vi "STS.vi"() -> ()   [LabVIEW 2014]
panel:
  out "Efficiency":dbl
  out "Mechanical Output Power":dbl
  out "Supply power":dbl
  out "Speed":dbl
  out "i":dbl
  in  "Supply Voltage":dbl
  in  "Load Torque":dbl
  # "Ahmed Adel Hassan Elmashhor"
  # "Sec 1"
  # "Steady State Analysis of DC Motor"
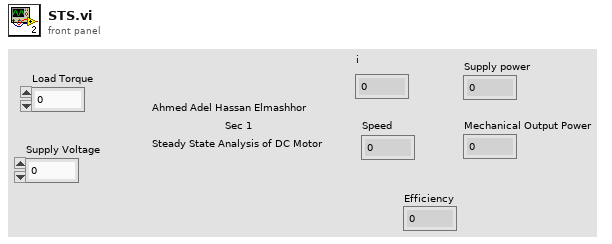
[diagram p1: front panel]
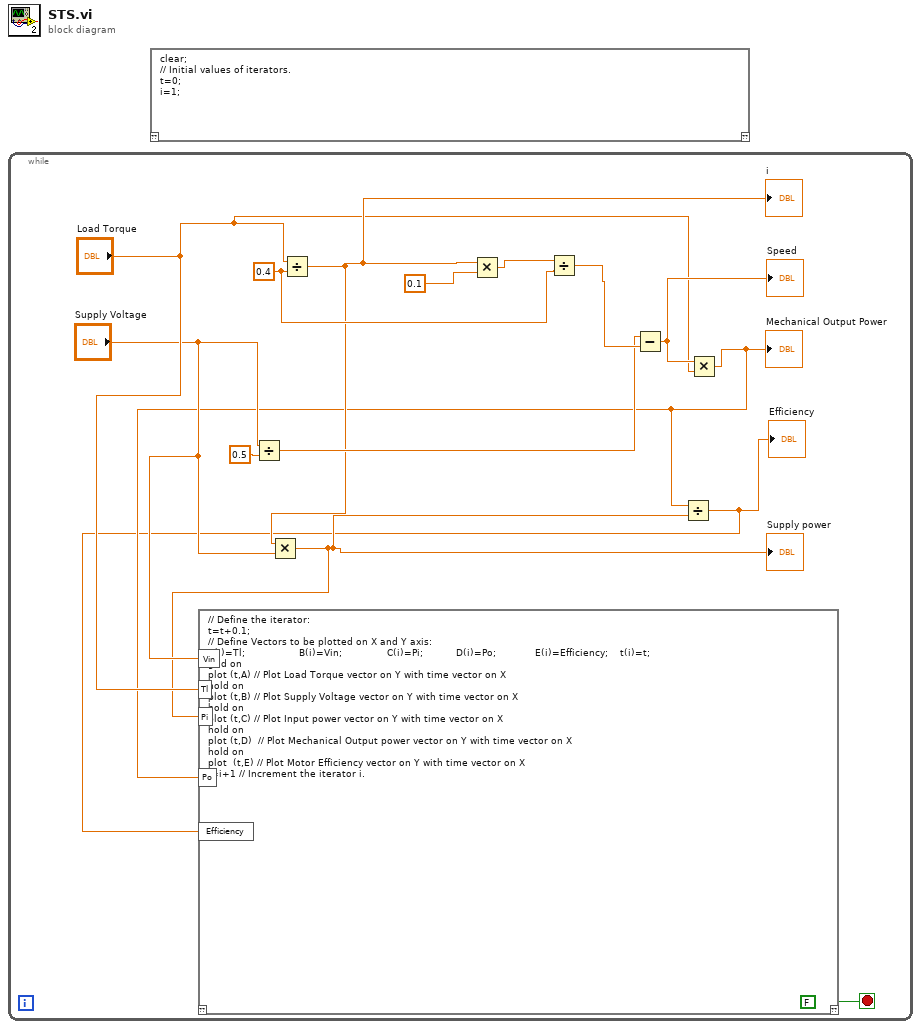
[diagram p0: block diagram]
diagram:
  n1 = while {
    stop <- FALSE stop-if-true
    w12 = 0.4 ("y")
    n2 = Divide(x="Supply Voltage", y=0.5) -> (x/y=w9:dbl)
    n3 = Divide(x="Load Torque", y=w12) -> (x/y=w8:dbl)
    "i" <- w8
    n4 = Multiply(x=w8, y="Supply Voltage") -> (x*y=w4:dbl)
    "Supply power" <- w4
    n5 = Multiply(x=w8, y=0.1) -> (x*y=w13:dbl)
    n6 = Divide(x=w13, y=w12) -> (x/y=w11:dbl)
    n7 = Subtract(x=w9, y=w11) -> (x-y=w7:dbl)
    "Speed" <- w7
    n8 = Multiply(x=w7, y="Load Torque") -> (x*y=w3:dbl)
    "Mechanical Output Power" <- w3
    n9 = Divide(x=w3, y=w4) -> (x/y=w2:dbl)
    "Efficiency" <- w2
    n10 = script code="// Define the iterator: \nt=t+0.1;   \n// Define Vectors to be plotted on X and Y axis:\nA(i)=Tl;                  B(i)=Vin;               C(i)=Pi;           D(i)=Po;             E(i)=Efficiency;    t(i)=t;\ngrid on\nplot (t,A) // Plot Load Torque vector on Y with time vector on X\nhold on\nplot (t,B) // Plot Supply Voltage vector on Y with time vector on X\nhold on\nplot (t,C) // Plot Input power vector on Y with time vector on X\nhold on\nplot (t,D)  // Plot Mechanical Output power vector on Y with time vector on X\nhold on\nplot  (t,E) // Plot Motor Efficiency vector on Y with time vector on X\ni=i+1 // Increment the iterator i."("Tl"="Load Torque", "Vin"="Supply Voltage", "Pi"=w4, "Po"=w3, "Efficiency"=w2) -> ()  [unwired: 1 in, 1 out]
  }
  n11 = script code="clear;\n// Initial values of iterators. \nt=0;\ni=1;"() -> ()  [unwired: 1 in, 1 out]
